vi "CleanFilename.vi"(6 "Clean Filename?":bool, 11 "Filename In":path) -> (3 "Filename out":path)   [LabVIEW 2022 SP3]
uses:
  <vilib>/Utility/error.llb/Trim Whitespace One-Sided.vi
  <userlib>/_OpenG.lib/file/file.llb/Strip Path Extension - String__ogtk.vi
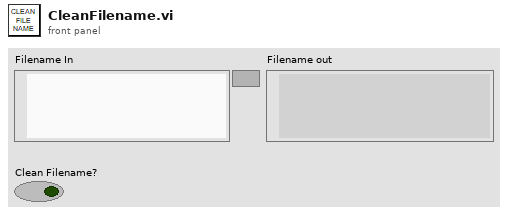
[diagram p1: front panel]
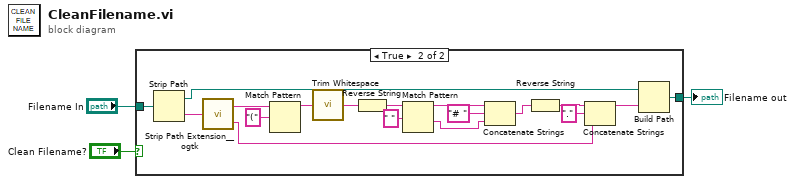
[diagram p0: block diagram]
diagram:
  n1 = case shown="True" "Clean Filename?" {
    tunnel: "Filename In" -> [w4 w22]
    tunnel: [w4 w16] -> w2
    frame False {
    }
    frame True {
      n2 = Strip Path(path=w22) -> (stripped path=w17:path, name=w21:string)
      n3 = call-poly <userlib>:"Strip Path Extension__ogtk.vi"("path"=w21) -> ("root"=w20:string, "extension"=w14:string)
      n4 = Match Pattern(string=w20, regular expression="(") -> (before substring=w18:string)  [unwired: 1 in, 3 out]
      n5 = call <vilib>:"Trim Whitespace.vi"("string"=w18) -> ("trimmed string"=w12:string)  [unwired: 1 in]
      n6 = Reverse String(1:w12) -> (0:w11:string)
      n7 = Match Pattern(string=w11, regular expression=" ") -> (before substring=w9:string, after substring=w7:string)  [unwired: 1 in, 2 out]
      n8 = Concatenate Strings(w9, "# " ("string"), w7) -> (w6:string)
      n9 = Reverse String(1:w6) -> (0:w5:string)
      n10 = Concatenate Strings(w5, "." ("string"), w14) -> (w15:string)
      n11 = Build Path(base path=w17, name or relative path=w15) -> (appended path=w16:path)
    }
  }
  "Filename out" <- w2
